vi "LoadCommands.vi"(11 "File":path) -> ()   [LabVIEW 2014]
uses:
  <vilib>/Utility/file.llb/Read From Spreadsheet File (DBL).vi
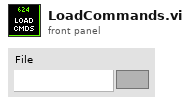
[diagram p1: front panel]
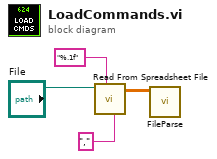
[diagram p0: block diagram]
diagram:
  n1 = call-poly <vilib>:"Read From Spreadsheet File.vi"("delimiter (\\t)"="," ("delimiter (\\t)"), "format (%.3f)"="%.1f", "file path (dialog if empty)"="File") -> ("all rows"=w1:dbl[][])  [unwired: 4 in, 4 out]
  n2 = call "FileParse.vi"("all rows"=w1) -> ()  [unwired: 10 in]
